vi "EIP_data reader.vi"() -> ()   [LabVIEW 2023]
doc: "Demonstrates how to read and set the attributes of Identity Object using Explicit Messaging."
uses:
  <vilib>/ethernetip/ethernetip.lvlib
panel:
  out "Array":sgl[](array[numeric])
  out "Data":u8[](array[numeric])
  in  "update rate [ms]":u32=500
  in  "stop":bool
  out "running?":bool
  in  "timeout [ms]":i32=1000
  in  "attribute":i32=15 format="%.0x"
  in  "instance":u32=1
  in  "class":i32=1 format="%.0x"
  in  "network path":string="*.*.*.*"
  # "Configuration"
  # "Original Attribute Values"
  # "Assign Attribute Values"
  # "Assigned Attribute Values"
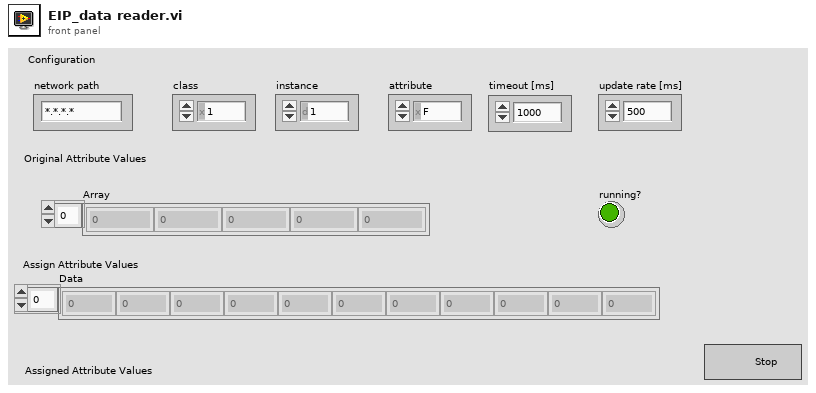
[diagram p1: front panel]
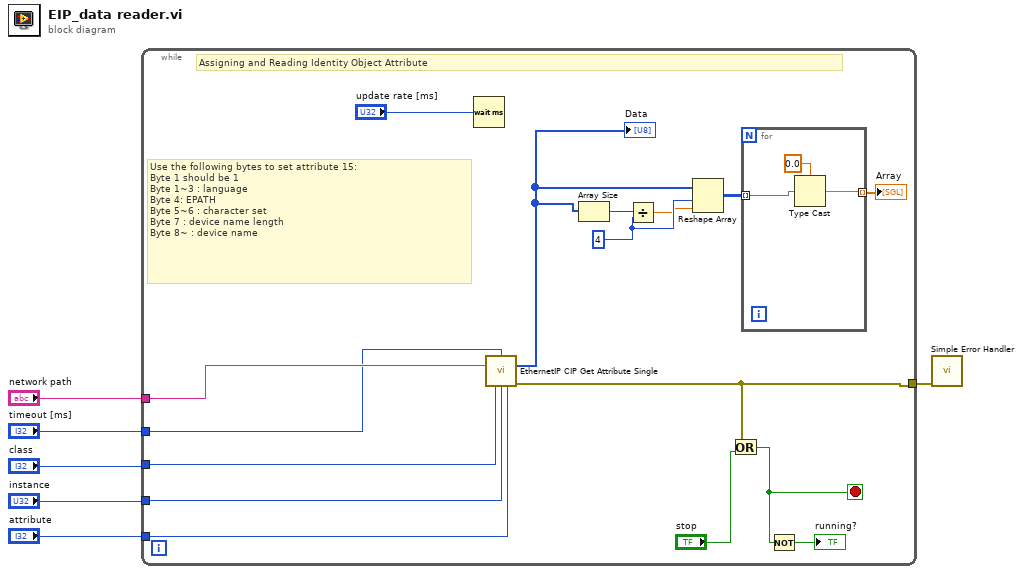
[diagram p0: block diagram]
diagram:
  n1 = while {
    tunnel: "network path" -> [w21]
    tunnel: "class" -> [w19]
    tunnel: "instance" -> [w18]
    tunnel: "attribute" -> [w16]
    tunnel: "timeout [ms]" -> [w20]
    tunnel: [w13] -> w1
    stop <- w15 stop-if-true
    w12 = 4
    # "Use the following bytes to set attribute 15:\nByte 1 should be 1\nByte 1~3 : language\nByte 4: EPATH\nByte 5~6 : character set\nByte 7 : device name length\nByte 8~ : device name"
    # "Assigning and Reading Identity Object Attribute"
    n2 = Wait (ms)(milliseconds to wait="update rate [ms]") -> ()  [unwired: 1 out]
    n3 = call <vilib>:"EthernetIP CIP Get Attribute Single.vi"("Timeout (ms)"=w20, "Network Path"=w21, "Class"=w19, "Instance"=w18, "Attribute"=w16) -> ("Data"=w10:u8[], "error out"=w13:errorcluster)  [unwired: 2 in, 7 out]
    "Data" <- w10
    n4 = Array Size(array=w10) -> (size(s)=w9:i32)
    n5 = Divide(x=w9, y=w12) -> (x/y=w11:dbl)
    n6 = Reshape Array(w10, w12, w11) -> (w8:u8[][])
    n7 = Or(x=w13, y="stop") -> (x .or. y?=w15:bool)
    n8 = for {
      tunnel: w8 -> [w24] mode=indexing
      tunnel: [w23] -> w7 mode=indexing
      n9 = Type Cast(type=sgl 0.0, x=w24) -> (*(type *) &x=w23:sgl)
    }
    "Array" <- w7
    n10 = Not(x=w15) -> (.not. x?=→"running?":bool)
  }
  n11 = call <vilib>:"Simple Error Handler.vi"("error in (no error)"=w1) -> ()  [unwired: 1 in, 8 out]
